vi "test_easy_lin_int_FFT.vi"() -> ()   [LabVIEW 2009]
doc: "Copyright (C) 2009, Stepan A. Baranov\nweb: http://www.OCTLab.org/\nemail: stepan@baranov.su"
uses:
  <vilib>/Analysis/4window.llb/Hanning Window (DBL).vi
  <vilib>/Analysis/NI_AALPro.lvlib
  OCTLib.dll
  <vilib>/gmath/NI_Gmath.lvlib
panel:
  out "error out":errorcluster
  out "Im part":dbl[](array[numeric])
  out "Re part":dbl[](array[numeric])
  out "Phase A-scan":dbl[](array[numeric])
  out "Intensity A-scan":dbl[](array[numeric])
  out "Im":dbl[](array[numeric])
  out "Re":dbl[](array[numeric])
  out "phase":dbl[](array[numeric])
  out "intensity":dbl[](array[numeric])
  out "time for FFT":u32
  in  "RSM_STAT?":bool=TRUE
  in  "stop":bool
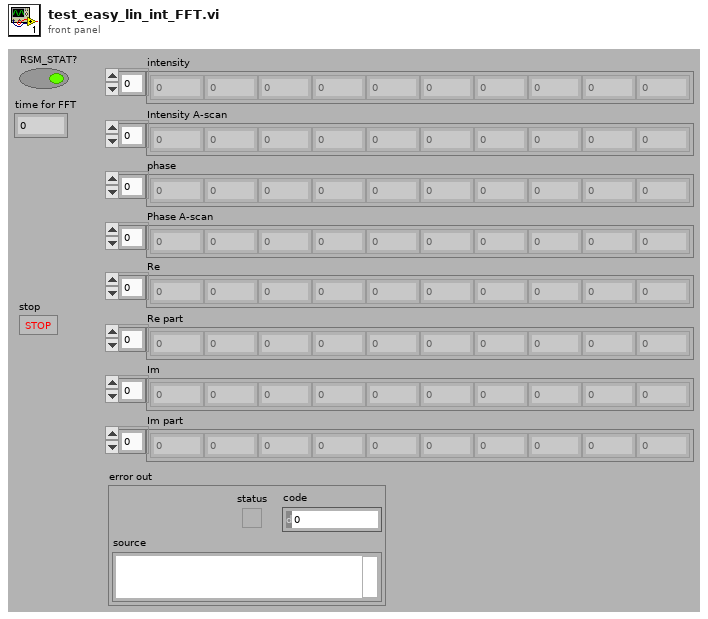
[diagram p1: front panel]
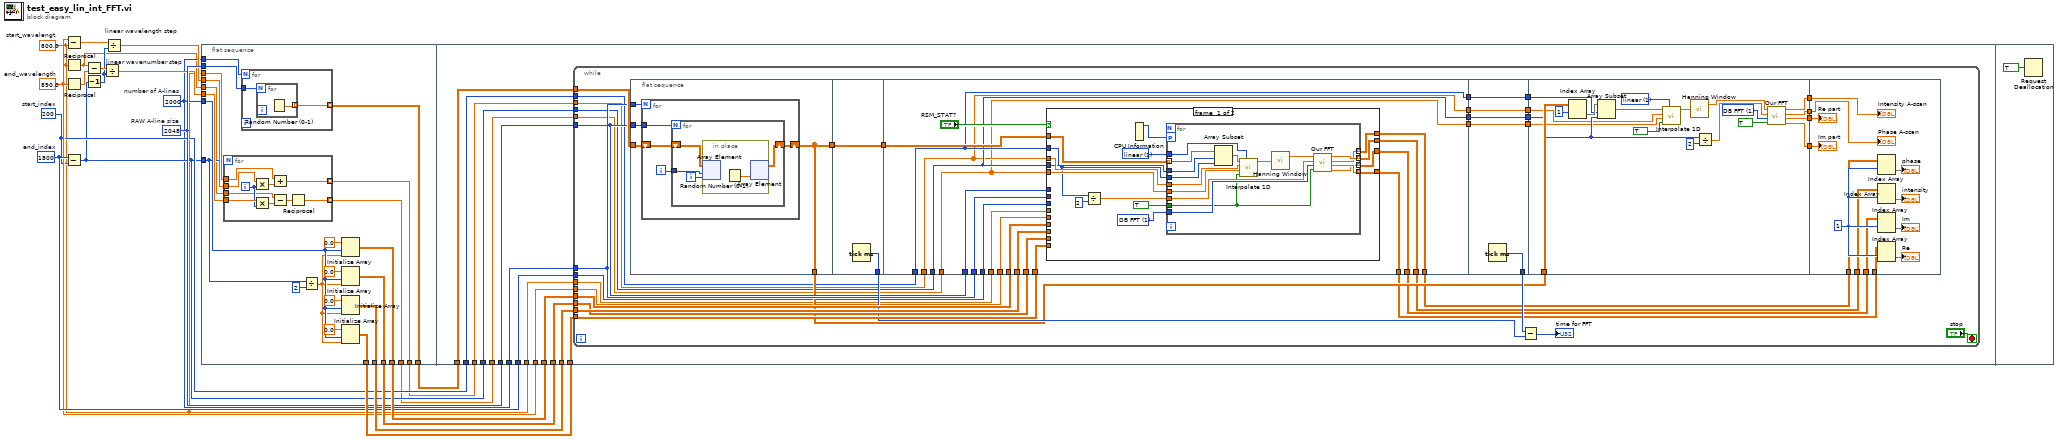
[diagram p0: block diagram]
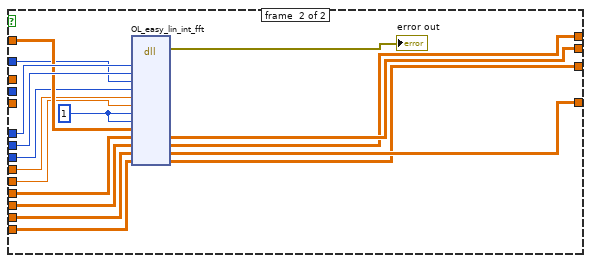
[diagram p2: hidden frame]
diagram:
  w1 = 800.0  # start_wavelengt
  w9 = 890.0  # end_wavelength
  w15 = 1800  # end_index
  w8 = 200  # start_index
  w4 = 2000  # number of A-lines
  w16 = 2048  # RAW A-line size
  n1 = Subtract(x=w9, y=w1) -> (x-y=w14:dbl)
  n2 = Reciprocal(x=w1) -> (1/x=w2:dbl)
  n3 = Reciprocal(x=w9) -> (1/x=w3:dbl)
  n4 = Subtract(x=w15, y=w8) -> (x-y=w7:i32)
  n5 = Subtract(x=w2, y=w3) -> (x-y=w13:dbl)
  n6 = Decrement(x=w7) -> (x-1=w12:i32)
  n7 = Divide "linear wavenumber step"(x=w13, y=w12) -> (x/y=w11:dbl)
  n8 = Divide "linear wavelength step"(x=w14, y=w12) -> (x/y=w10:dbl)
  n9 = flat-sequence {
    tunnel: w16 -> [w42]
    tunnel: w4 -> [w41]
    tunnel: w4 -> [w36]
    tunnel: [w35] -> w21
    tunnel: [w34] -> w20
    tunnel: [w33] -> w19
    tunnel: [w32] -> w18
    tunnel: [w31] -> w17
    tunnel: w7 -> [w25]
    tunnel: w11 -> [w30]
    tunnel: w10 -> [w29]
    tunnel: w1 -> [w28]
    tunnel: [w27] -> w6
    tunnel: [w26] -> w5
    tunnel: w2 -> [w22]
    tunnel: w4 -> [w69]
    tunnel: w16 -> [w68]
    tunnel: w21 -> [w67]
    tunnel: w20 -> [w66]
    tunnel: w19 -> [w65]
    tunnel: w18 -> [w64]
    tunnel: w17 -> [w63]
    tunnel: w8 -> [w62]
    tunnel: w15 -> [w61]
    tunnel: w1 -> [w60]
    tunnel: w9 -> [w59]
    tunnel: w7 -> [w58]
    tunnel: w6 -> [w57]
    tunnel: w5 -> [w56]
    frame #0 {
      n10 = for {
        N: w25 -> [_]
        tunnel: w30 -> [w52]
        tunnel: [w44] -> w26 mode=indexing
        tunnel: w29 -> [w49]
        tunnel: w28 -> [w48]
        tunnel: [w43] -> w27 mode=indexing
        tunnel: w22 -> [w46]
        i -> [w50]
        n11 = Multiply(x=w49, y=w50) -> (x*y=w47:dbl)
        n12 = Multiply(x=w52, y=w50) -> (x*y=w51:dbl)
        n13 = Add(x=w48, y=w47) -> (x+y=w43:dbl)
        n14 = Subtract(x=w46, y=w51) -> (x-y=w45:dbl)
        n15 = Reciprocal(x=w45) -> (1/x=w44:dbl)
      }
      n16 = for {
        N: w41 -> [_]
        tunnel: [w54] -> w31 mode=indexing
        tunnel: w42 -> [w53]
        n17 = for {
          N: w53 -> [_]
          tunnel: [w55] -> w54 mode=indexing
          n18 = Random Number (0-1)() -> (number: 0 to 1=w55:dbl)
        }
      }
      n19 = Divide(x=w25, y=2) -> (x/y=w23:dbl)
      n20 = Initialize Array(0.0 ("element"), w36, w23) -> (w34:dbl[][])
      n21 = Initialize Array(0.0 ("element"), w36, w23) -> (w33:dbl[][])
      n22 = Initialize Array(0.0 ("element"), w36, w23) -> (w35:dbl[][])
      n23 = Initialize Array(0.0 ("element"), w36, w23) -> (w32:dbl[][])
    }
    frame #1 {
      n24 = while {
        tunnel: w63 -> [w105]
        tunnel: w69 -> [w97]
        tunnel: w68 -> [w96]
        tunnel: w67 -> [w104]
        tunnel: w66 -> [w103]
        tunnel: w65 -> [w102]
        tunnel: w64 -> [w101]
        tunnel: w62 -> [w84]
        tunnel: w61 -> [w83]
        tunnel: w60 -> [w82]
        tunnel: w59 -> [w81]
        tunnel: w58 -> [w80]
        tunnel: w57 -> [w79]
        tunnel: w56 -> [w78]
        stop <- "stop" stop-if-true
        n25 = flat-sequence {
          tunnel: w105 -> [w110]
          tunnel: w97 -> [w109]
          tunnel: w96 -> [w108]
          tunnel: [w107] -> w95
          tunnel: [w107] -> w85
          tunnel: [w121] -> w100
          tunnel: [w120] -> w86
          tunnel: w85 -> [w120]
          tunnel: w104 -> [w139]
          tunnel: w103 -> [w138]
          tunnel: w102 -> [w137]
          tunnel: w101 -> [w136]
          tunnel: w96 -> [w135]
          tunnel: w97 -> [w134]
          tunnel: [w133] -> w90
          tunnel: [w132] -> w89
          tunnel: [w131] -> w88
          tunnel: [w130] -> w87
          tunnel: w86 -> [w129]
          tunnel: w84 -> [w125]
          tunnel: w83 -> [w128]
          tunnel: w82 -> [w127]
          tunnel: w81 -> [w126]
          tunnel: w80 -> [w124]
          tunnel: w79 -> [w123]
          tunnel: w78 -> [w122]
          tunnel: [w125] -> w76
          tunnel: [w124] -> w74
          tunnel: [w123] -> w73
          tunnel: [w122] -> w70
          tunnel: [w193] -> w98
          tunnel: [w192] -> w77
          tunnel: w76 -> [w192]
          tunnel: [w191] -> w75
          tunnel: w74 -> [w191]
          tunnel: w73 -> [w190]
          tunnel: [w190] -> w72
          tunnel: [w189] -> w71
          tunnel: w70 -> [w189]
          tunnel: w95 -> [w213]
          tunnel: [w208] -> w94
          tunnel: [w207] -> w93
          tunnel: [w206] -> w92
          tunnel: [w205] -> w91
          tunnel: w77 -> [w203]
          tunnel: w75 -> [w202]
          tunnel: w72 -> [w196]
          tunnel: w71 -> [w195]
          tunnel: w94 -> [w226]
          tunnel: w93 -> [w225]
          tunnel: w92 -> [w224]
          tunnel: w91 -> [w223]
          tunnel: w90 -> [w221]
          tunnel: w89 -> [w219]
          tunnel: w88 -> [w217]
          tunnel: w87 -> [w215]
          frame #0 {
            n26 = for {
              N: w109 -> [_]
              shift-right: [w112] -> w107
              shift-left: w110 -> [w113]
              tunnel: w108 -> [w114]
              i -> [w111]
              n27 = for {
                N: w114 -> [_]
                shift-right: [w115] -> w112
                shift-left: w113 -> [w118]
                tunnel: w111 -> [w117]
                i -> [w116]
                n28 = in-place {
                  n29 = in-place-array #1(w118, w117, w116) -> ()  [unwired: 1 out]
                  n30 = Random Number (0-1)() -> (number: 0 to 1=w119:dbl)
                  n31 = in-place-array #1(w119) -> (w115:dbl[][])  [unwired: 2 out]
                }
              }
            }
          }
          frame #1 {
            n32 = Tick Count (ms)() -> (millisecond timer value=w121:u32)
          }
          frame #2 {
            n33 = case shown="True" "RSM_STAT?" {
              tunnel: w139 -> [_ w185]
              tunnel: w138 -> [_ w188]
              tunnel: w137 -> [_ w187]
              tunnel: w136 -> [_ w186]
              tunnel: w135 -> [_ w184]
              tunnel: w134 -> [_ w183]
              tunnel: w129 -> [w155 w181]
              tunnel: [w151 w180] -> w133
              tunnel: [w150 w179] -> w132
              tunnel: [w149 w178] -> w131
              tunnel: [w148 w177] -> w130
              tunnel: w125 -> [w147 w176]
              tunnel: w128 -> [_ w175]
              tunnel: w127 -> [_ w174]
              tunnel: w126 -> [_ w173]
              tunnel: w124 -> [w144 _]
              tunnel: w123 -> [w146 _]
              tunnel: w122 -> [w145 _]
              frame #0 {
                w141 = 1 items=["nearest", "linear", "spline", "cubic Hermite", "Lagrange"] ("method")
                w152 = 1 items=["LINEAR FFT", "DB FFT"] ("A-scan type")
                n34 = Divide(x=w144, y=2) -> (x/y=w142:dbl)
                n35 = CPU Information() -> (4:w154:i32)  [unwired: 3 out]
                n36 = for {
                  workers-P: w154 -> [_]
                  tunnel: [w170] -> w151 mode=indexing
                  tunnel: [w169] -> w150 mode=indexing
                  tunnel: [w168] -> w149 mode=indexing
                  tunnel: [w167] -> w148 mode=indexing
                  tunnel: w155 -> [w165] mode=indexing
                  tunnel: TRUE ("need phase?") -> [w156]
                  tunnel: w152 -> [w166]
                  tunnel: w147 -> [w164]
                  tunnel: w144 -> [w163]
                  tunnel: w146 -> [w159]
                  tunnel: w145 -> [w158]
                  tunnel: w142 -> [w162]
                  tunnel: w141 -> [w161]
                  n37 = Array Subset(array=w165, index=w164, length=w163) -> (w160:dbl[])
                  n38 = call <vilib>:"Interpolate 1D.vi"("method"=w161, "X is monotonic"=w156, "xi"=w158, "X"=w159, "Y"=w160) -> ("yi"=w157:dbl[])  [unwired: 4 in, 2 out]
                  n39 = call-poly <vilib>:"Hanning Window.vi"("X"=w157) -> ("Windowed X"=w171:dbl[])  [unwired: 1 out]
                  n40 = call "Our FFT.vi"("need phase?"=w156, "A-scan type"=w166, "FFT A-scan size"=w162, "RAW A-line"=w171) -> ("Im part"=w167:dbl[], "Re part"=w168:dbl[], "Phase A-scan"=w169:dbl[], "Intensity A-scan"=w170:dbl[])
                }
              }
              frame #1 {
                w182 = i8 1 ("hanning_flag")
                n41 = dll-call lib="OCTLib.dll" fn="OL_easy_lin_int_fft"("width"=w184, "height"=w183, "start_index"=w176, "end_index"=w175, "start_wavelengt"=w174, "end_wavelength"=w173, "hanning_flag"=w182, "log10_flag"=w182, "input"=w181, "intensity"=w188, "phase"=w187, "Re"=w185, "Im"=w186) -> (error out=→"error out":errorcluster, "intensity"=w180:dbl[][], "phase"=w179:dbl[][], "Re"=w178:dbl[][], "Im"=w177:dbl[][])  [unwired: 13 in, 1 out]
              }
            }
          }
          frame #3 {
            n42 = Tick Count (ms)() -> (millisecond timer value=w193:u32)
          }
          frame #4 {
            w198 = 1 items=["nearest", "linear", "spline", "cubic Hermite", "Lagrange"] ("method")
            w210 = 1 items=["LINEAR FFT", "DB FFT"] ("A-scan type")
            n43 = Index Array(array=w213, index (row)=1) -> (element=w204:dbl[])  [unwired: 1 in]
            n44 = Array Subset(array=w204, index=w203, length=w202) -> (w197:dbl[])
            n45 = call <vilib>:"Interpolate 1D.vi"("method"=w198, "X is monotonic"=TRUE, "xi"=w195, "X"=w196, "Y"=w197) -> ("yi"=w194:dbl[])  [unwired: 4 in, 2 out]
            n46 = call-poly <vilib>:"Hanning Window.vi"("X"=w194) -> ("Windowed X"=w211:dbl[])  [unwired: 1 out]
            n47 = Divide(x=w202, y=2) -> (x/y=w200:dbl)
            n48 = call "Our FFT.vi"("need phase?"=TRUE, "A-scan type"=w210, "FFT A-scan size"=w200, "RAW A-line"=w211) -> ("Im part"=w205:dbl[], "Re part"=w206:dbl[], "Phase A-scan"=w207:dbl[], "Intensity A-scan"=w208:dbl[])
          }
          frame #5 {
            w222 = 1 ("index (row)")
            n49 = Index Array(array=w219, index (row)=w222) -> (element=→"phase":dbl[])  [unwired: 1 in]
            n50 = Index Array(array=w221, index (row)=w222) -> (element=→"intensity":dbl[])  [unwired: 1 in]
            n51 = Index Array(array=w215, index (row)=w222) -> (element=→"Im":dbl[])  [unwired: 1 in]
            n52 = Index Array(array=w217, index (row)=w222) -> (element=→"Re":dbl[])  [unwired: 1 in]
            "Intensity A-scan" <- w226
            "Phase A-scan" <- w225
            "Re part" <- w224
            "Im part" <- w223
          }
        }
        n53 = Subtract(x=w98, y=w100) -> (x-y=→"time for FFT":u32)
      }
    }
    frame #2 {
      n54 = Request Deallocation(TRUE ("flag")) -> ()
    }
  }
